vi "mClampAxon2A.vi"() -> ()   [LabVIEW 2011]
uses:
  <vilib>/DAQmx/write.llb/DAQmx Write (Analog Wfm 1Chan NSamp).vi
  <vilib>/DAQmx/read.llb/DAQmx Read (Analog 1D Wfm NChan NSamp).vi
  <vilib>/DAQmx/create/channels.llb/DAQmx Create Channel (AO-Voltage-Basic).vi
  <vilib>/DAQmx/configure/timing.llb/DAQmx Timing (Sample Clock).vi
  <vilib>/DAQmx/create/channels.llb/DAQmx Create Channel (AI-Voltage-Basic).vi
  <vilib>/DAQmx/miscellaneous.llb/DAQmx Fill In Error Info.vi
  <vilib>/ptbypt/NI_PtbyPt.lvlib
panel:
  out "reversed array":i32[](array[numeric])
  out "Waveform Graph":dynamicdata(graph)
  out "refresh":bool
  in  "Amplitude (nA)":dbl=2.0
  out "Waveform Chart":dynamicdata(graph)
  in  "Voltage Clamp":bool=TRUE
  out "Resistance (MOhm)":dbl
  out "Off":bool
  out "On":bool
  in  "Amplitude (mV)":dbl=10.0
  in  "R test":bool
  in  "Off Time (msec)":u32=1000
  in  "On Time (msec)":u32=100
  in  "stop":bool
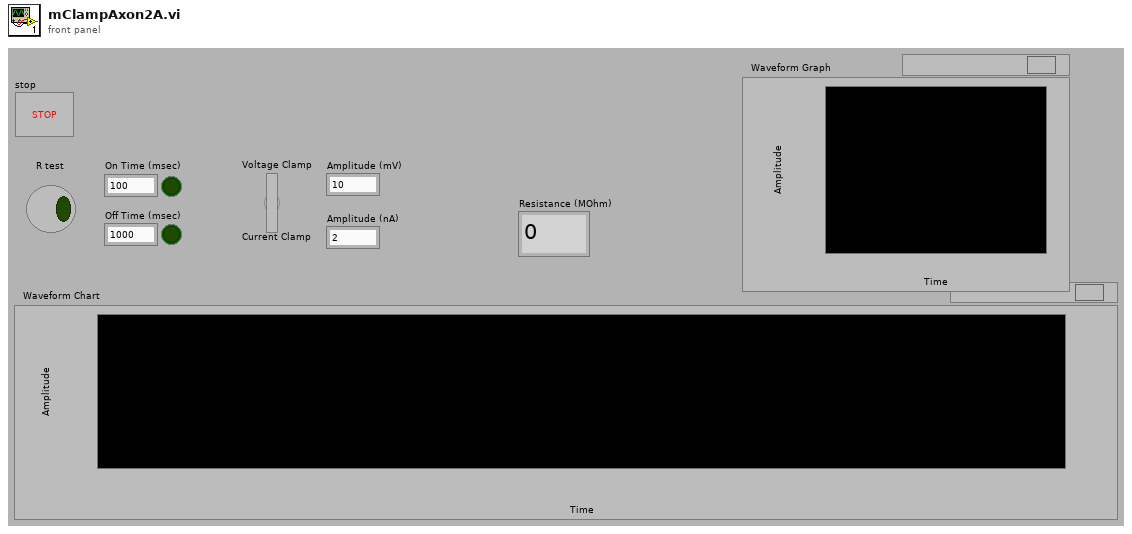
[diagram p1: front panel]
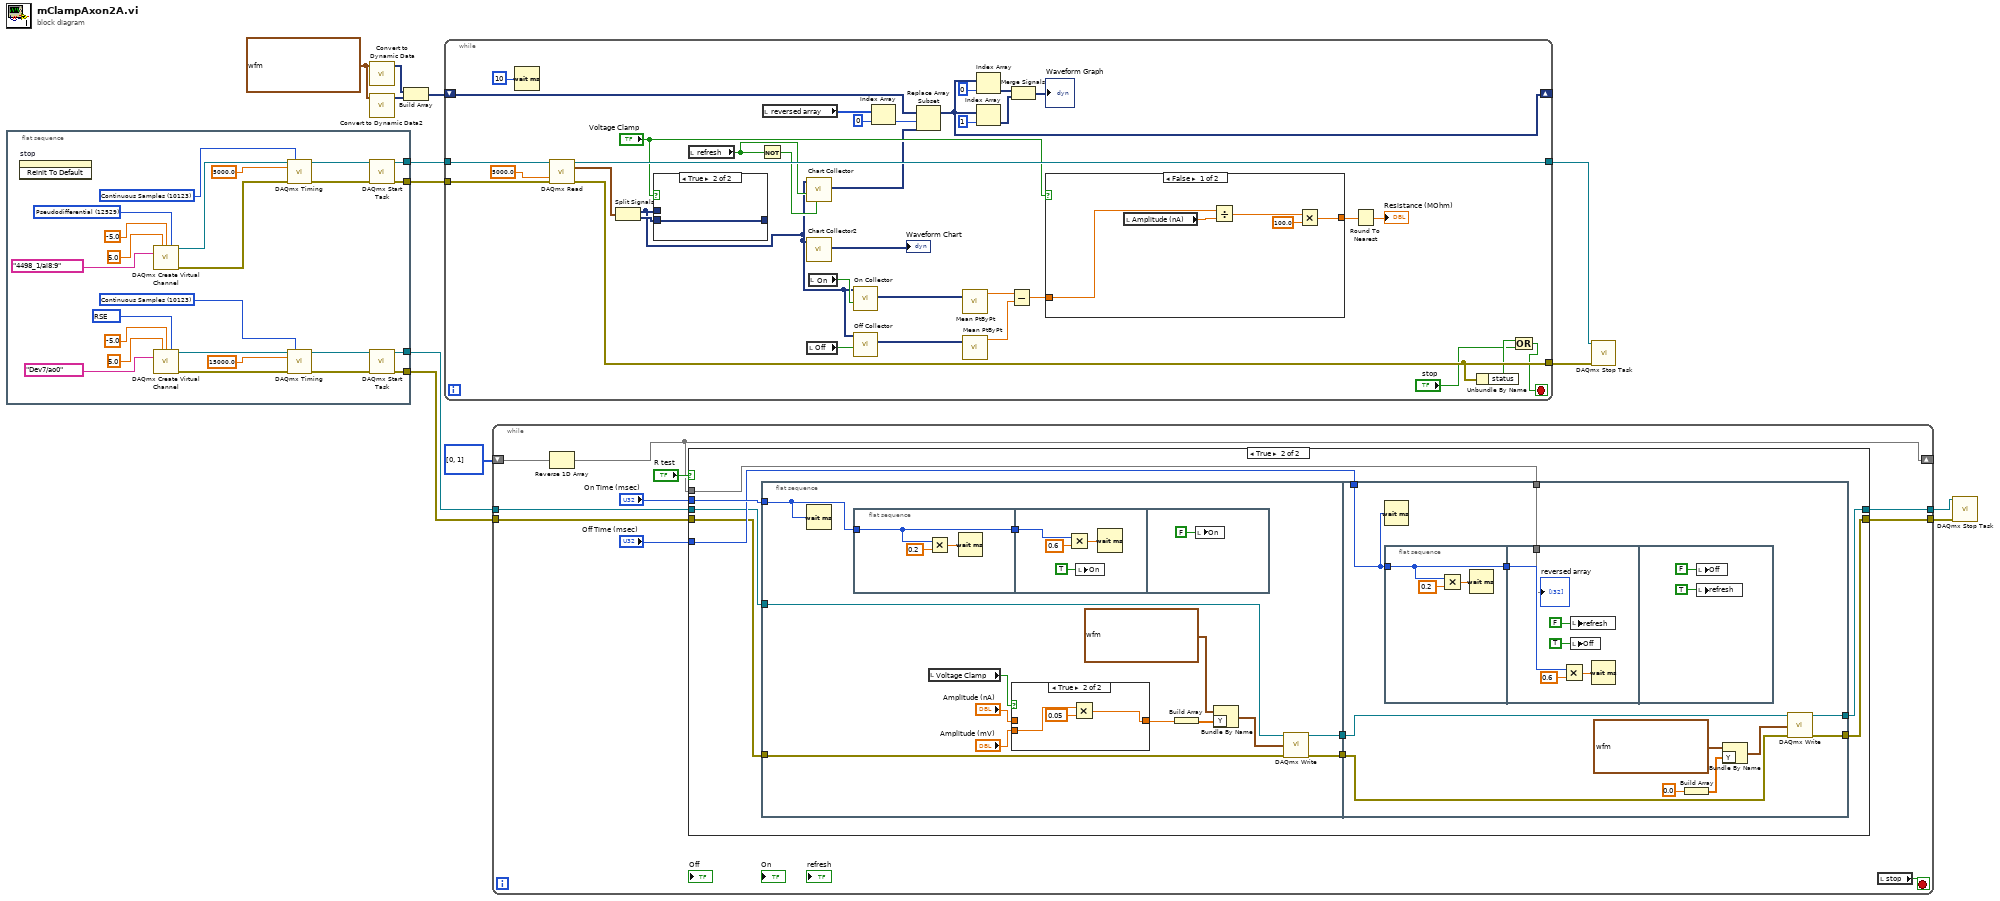
[diagram p0: block diagram]
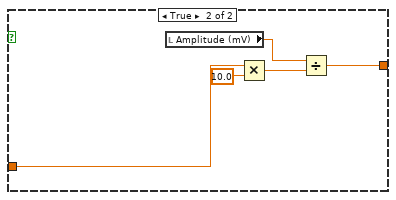
[diagram p4: hidden frame]
diagram:
  w5 = waveform(dbl) {"t0"=timestamp(0 s since 1904-01-01), "dt"=1.0, "Y"=[]} ("Waveform")
  n1 = flat-sequence {
    tunnel: [w29] -> w13
    tunnel: [w28] -> w12
    tunnel: [w15] -> w9
    tunnel: [w14] -> w8
    frame #0 {
      w25 = 10083 items=["default"=-1, "RSE"=10083, "NRSE"=10078, "Differential"=10106, "Pseudodifferential"=12529] ("input terminal configuration")
      w21 = 10123 items=["Finite Samples"=10178, "Continuous Samples"=10123, "Hardware Timed Single Point"=12522] ("sample mode")
      w26 = 12529 items=["default"=-1, "RSE"=10083, "NRSE"=10078, "Differential"=10106, "Pseudodifferential"=12529] ("input terminal configuration")
      w33 = 10123 items=["Finite Samples"=10178, "Continuous Samples"=10123, "Hardware Timed Single Point"=12522] ("sample mode")
      n2 = invoke on="stop" class="Bool (strict)" method="Reinit To Default"() -> ()  [unwired: 3 in, 3 out]
      n3 = call-poly <vilib>:"DAQmx Create Virtual Channel.vi"("maximum value"=5.0, "minimum value"=-5.0, "input terminal configuration"=w26, "physical channels"=tag "4498_1/ai8:9") -> ("task out"=w35:refnum<k21>, "error out"=w34:errorcluster)  [unwired: 10 in]
      n4 = call-poly <vilib>:"DAQmx Create Virtual Channel.vi"("maximum value"=5.0, "minimum value"=-5.0, "output terminal configuration"=w25, "physical channels"=tag "Dev7/ao0" ("physical channels 2")) -> ("task out"=w19:refnum<k21>, "error out"=w20:errorcluster)  [unwired: 10 in]
      n5 = call-poly <vilib>:"DAQmx Timing.vi"("task/channels in"=w35, "sample mode"=w33, "rate"=5000.0, "error in"=w34) -> ("task out"=w37:refnum<k21>, "error out"=w36:errorcluster)  [unwired: 10 in]
      n6 = call-poly <vilib>:"DAQmx Timing.vi"("task/channels in"=w19, "sample mode"=w21, "rate"=15000.0, "error in"=w20) -> ("task out"=w17:refnum<k21>, "error out"=w18:errorcluster)  [unwired: 10 in]
      n7 = call <vilib>:"DAQmx Start Task.vi"("task/channels in"=w37, "error in"=w36) -> ("task out"=w29:refnum<k21>, "error out"=w28:errorcluster)  [unwired: 12 in]
      n8 = call <vilib>:"DAQmx Start Task.vi"("task/channels in"=w17, "error in"=w18) -> ("task out"=w15:refnum<k21>, "error out"=w14:errorcluster)  [unwired: 12 in]
    }
  }
  n9 = call "Convert to Dynamic Data"("Waveform"=w5) -> ("Dynamic Data Type"=w3:dynamicdata)  [unwired: 3 in]
  n10 = call "Convert to Dynamic Data2"("Waveform"=w5) -> ("Dynamic Data Type"=w4:dynamicdata)  [unwired: 3 in]
  n11 = Build Array(w3, w4) -> (w2:dynamicdata[])
  n12 = while {
    tunnel: w13 -> [w71]
    tunnel: w12 -> [w70]
    tunnel: [w69] -> w7
    tunnel: [w42] -> w6
    shift-right: [w45] -> _
    shift-left: w2 -> [w49]
    stop <- w39 stop-if-true
    n13 = Wait (ms)(milliseconds to wait=u32 10) -> ()  [unwired: 1 out]
    n14 = call-poly <vilib>:"DAQmx Read.vi"("task/channels in"=w71, "timeout"=5000.0, "error in"=w70) -> ("task out"=w69:refnum<k21>, "data"=w68:waveform(dbl)[], "error out"=w42:errorcluster)  [unwired: 10 in]
    n15 = Split Signals(w68) -> (w38:dynamicdata, w65:dynamicdata)  [unwired: 2 in]
    n16 = case shown="True" "Voltage Clamp" {
      tunnel: w38 -> [w84 _]
      tunnel: w65 -> [_ w85]
      tunnel: [w84 w85] -> _
      frame False {
      }
      frame True {
      }
    }
    n17 = local read "refresh"() -> (w56:bool)
    n18 = Not(x=w56) -> (.not. x?=w55:bool)
    n19 = local read "reversed array"() -> (w48:i32[])
    n20 = call "Chart Collector"("Reset"=w55, "Enable"=w56, "Signals"=w38) -> ("Collected Signals"=w54:dynamicdata)  [unwired: 7 in, 1 out]
    n21 = call "Chart Collector2"("Signals"=w38) -> ("Collected Signals"=→"Waveform Chart":dynamicdata)  [unwired: 9 in, 1 out]
    n22 = local read "Off"() -> (w63:bool)
    n23 = local read "On"() -> (w64:bool)
    n24 = call "On Collector"("Enable"=w64, "Signals"=w38) -> ("Collected Signals"=w62:dynamicdata)  [unwired: 8 in, 1 out]
    n25 = call "Off Collector"("Enable"=w63, "Signals"=w38) -> ("Collected Signals"=w61:dynamicdata)  [unwired: 8 in, 1 out]
    n26 = Index Array(array=w48, index=0) -> (element=w46:i32)
    n27 = Replace Array Subset(array=w49, new element=w54, index=w46) -> (w45:dynamicdata[])
    n28 = call <vilib>:"Mean PtByPt.vi"("x"=w62) -> ("mean"=w60:dbl)  [unwired: 3 in, 1 out]
    n29 = call <vilib>:"Mean PtByPt.vi"("x"=w61) -> ("mean"=w59:dbl)  [unwired: 3 in, 1 out]
    n30 = Index Array(array=w45, index=0) -> (element=w53:dynamicdata)
    n31 = Index Array(array=w45, index=1) -> (element=w52:dynamicdata)
    n32 = Subtract(x=w60, y=w59) -> (x-y=w58:dbl)
    n33 = Merge Signals(w53, w52) -> (→"Waveform Graph":dynamicdata)
    n34 = case shown="False" "Voltage Clamp" {
      tunnel: w58 -> [w75 w80]
      tunnel: [w74 w79] -> w57
      frame False {
        n35 = local read "Amplitude (nA)"() -> (w76:dbl)
        n36 = Divide(x=w75, y=w76) -> (x/y=w77:dbl)
        n37 = Multiply(x=w77, y=100.0) -> (x*y=w74:dbl)
      }
      frame True {
        n38 = local read "Amplitude (mV)"() -> (w83:dbl)
        n39 = Multiply(x=w80, y=10.0) -> (x*y=w82:dbl)
        n40 = Divide(x=w83, y=w82) -> (x/y=w79:dbl)
      }
    }
    n41 = Round To Nearest(number=w57) -> (nearest integer value=→"Resistance (MOhm)":dbl)
    n42 = Unbundle By Name(w42) -> ("status"=w41:bool)
    n43 = Or(x=w41, y="stop") -> (x .or. y?=w39:bool)
  }
  n44 = while {
    tunnel: [w94] -> w11
    tunnel: [w88] -> w10
    tunnel: w9 -> [w90]
    tunnel: w8 -> [w89]
    shift-right: [w86] -> _
    shift-left: i32[] [0, 1] -> [w87]
    stop <- w95 stop-if-true
    n45 = Reverse 1D Array(array=w87) -> (reversed array=w86:i32[])
    n46 = case shown="True" "R test" {
      tunnel: [w97 w104] -> w94
      tunnel: "On Time (msec)" -> [_ w103]
      tunnel: "Off Time (msec)" -> [_ w102]
      tunnel: w90 -> [w97 w101]
      tunnel: w89 -> [w96 w100]
      tunnel: [w96 w99] -> w88
      tunnel: w86 -> [_ w98]
      frame False {
      }
      frame True {
        n47 = flat-sequence {
          tunnel: [w119] -> w106
          tunnel: [w118] -> w105
          tunnel: w103 -> [w115]
          tunnel: w101 -> [w114]
          tunnel: w100 -> [w113]
          tunnel: w106 -> [w142]
          tunnel: w105 -> [w141]
          tunnel: [w140] -> w104
          tunnel: [w139] -> w99
          tunnel: w102 -> [w135]
          tunnel: w98 -> [w132]
          frame #0 {
            n48 = Wait (ms)(milliseconds to wait=w115) -> ()  [unwired: 1 out]
            n49 = flat-sequence {
              tunnel: w115 -> [w124]
              tunnel: [w124] -> w116
              tunnel: w116 -> [w127]
              frame #0 {
                n50 = Multiply(x=w124, y=0.2) -> (x*y=w126:dbl)
                n51 = Wait (ms)(milliseconds to wait=w126) -> ()  [unwired: 1 out]
              }
              frame #1 {
                n52 = Multiply(x=w127, y=0.6) -> (x*y=w128:dbl)
                n53 = local write "On"(TRUE) -> ()
                n54 = Wait (ms)(milliseconds to wait=w128) -> ()  [unwired: 1 out]
              }
              frame #2 {
                n55 = local write "On"(FALSE ("Detect")) -> ()
              }
            }
            n56 = local read "Voltage Clamp"() -> (w107:bool)
            n57 = case shown="True" w107 {
              tunnel: [w120 w122] -> w110
              tunnel: "Amplitude (mV)" -> [_ w123]
              tunnel: "Amplitude (nA)" -> [w120 _]
              frame False {
              }
              frame True {
                n58 = Multiply(x=w123, y=0.05) -> (x*y=w122:dbl)
              }
            }
            n59 = Build Array(w110) -> (w117:dbl[])
            n60 = Bundle By Name(cluster=waveform(dbl) {"t0"=timestamp(0 s since 1904-01-01), "dt"=1.0, "Y"=[]} ("Waveform"), "Y"=w117) -> (w111:waveform(dbl))
            n61 = call-poly <vilib>:"DAQmx Write.vi"("task/channels in"=w114, "data"=w111, "error in"=w113) -> ("task out"=w119:refnum<k21>, "error out"=w118:errorcluster)  [unwired: 10 in, 1 out]
          }
          frame #1 {
            n62 = Wait (ms)(milliseconds to wait=w135) -> ()  [unwired: 1 out]
            n63 = flat-sequence {
              tunnel: w135 -> [w143]
              tunnel: [w143] -> w136
              tunnel: w136 -> [w148]
              tunnel: w132 -> [w146]
              frame #0 {
                n64 = Multiply(x=w143, y=0.2) -> (x*y=w145:dbl)
                n65 = Wait (ms)(milliseconds to wait=w145) -> ()  [unwired: 1 out]
              }
              frame #1 {
                n66 = Multiply(x=w148, y=0.6) -> (x*y=w149:dbl)
                n67 = local write "refresh"(FALSE ("refresh")) -> ()
                n68 = local write "Off"(TRUE) -> ()
                n69 = Wait (ms)(milliseconds to wait=w149) -> ()  [unwired: 1 out]
                "reversed array" <- w146
              }
              frame #2 {
                n70 = local write "Off"(FALSE ("Detect")) -> ()
                n71 = local write "refresh"(TRUE ("refresh")) -> ()
              }
            }
            n72 = Build Array(0.0) -> (w137:dbl[])
            n73 = Bundle By Name(cluster=waveform(dbl) {"t0"=timestamp(0 s since 1904-01-01), "dt"=1.0, "Y"=[]} ("Waveform"), "Y"=w137) -> (w133:waveform(dbl))
            n74 = call-poly <vilib>:"DAQmx Write.vi"("task/channels in"=w142, "data"=w133, "error in"=w141) -> ("task out"=w140:refnum<k21>, "error out"=w139:errorcluster)  [unwired: 10 in, 1 out]
          }
        }
      }
    }
    n75 = local read "stop"() -> (w95:bool)
  }
  n76 = call <vilib>:"DAQmx Stop Task.vi"("task/channels in"=w7, "error in"=w6) -> ()  [unwired: 12 in, 2 out]
  n77 = call <vilib>:"DAQmx Stop Task.vi"("task/channels in"=w11, "error in"=w10) -> ()  [unwired: 12 in, 2 out]
